vi "sedSpectrometer_getNextSample_LoopTimems.vi"(8 "error in (no error)":errorcluster, 11 "LoopTime_ms_Ctl":T1) -> (0 "error out":errorcluster, 2 "function return":i32, 3 "LoopTime_ms_Ctl out":T1)   [LabVIEW 2016, in "SALLV_sedSpectrometer.lvlib"]
doc: "int sedSpectrometer_shm_getNextSample_LoopTime_msLV(sedSpectrometer_LoopTime_msLV *LoopTime_ms_Ctl );"
uses:
  SALLV_sedSpectrometer.lvlib
  DataTypes/LoopTime_ms.ctl
  SALLV_sedSpectrometer.so
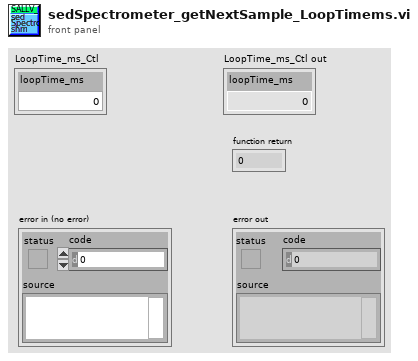
[diagram p1: front panel]
types:
  T1 = typedef "SALLV_sedSpectrometer.lvlib/LoopTime_ms.ctl" = cluster{"loopTime_ms":dbl}
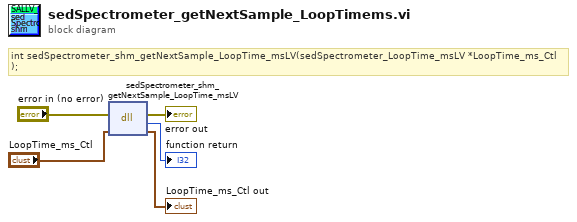
[diagram p0: block diagram]
diagram:
  # "int sedSpectrometer_shm_getNextSample_LoopTime_msLV(sedSpectrometer_LoopTime_msLV *LoopTime_ms_Ctl );"
  n1 = dll-call lib="home/harini/TCS/sallv_sedSpectrometer/SALLV_sedSpectrometer.*" fn="sedSpectrometer_shm_getNextSample_LoopTime_msLV"(error in="error in (no error)", "LoopTime_ms_Ctl"="LoopTime_ms_Ctl") -> (error out=→"error out":errorcluster, →"function return":i32, "LoopTime_ms_Ctl"=→"LoopTime_ms_Ctl out":T1)  [unwired: 2 in, 1 out]
